vi "broadRvsTp.vi"(2 "# points":dbl=1023.0 format="%.2f", 3 "R_offset":dbl format="%.3f", 4 "Delta T":dbl=1.15 format="%.3f", 5 "T mean":dbl=2.35 format="%.3f", 6 "T max":dbl=12.0 format="%.2f", 7 "T min":dbl format="%.2f", 8 "n norm?":u8=7, 9 "?":dbl[][](array[numeric])=[[0.478, 1.52], [0.813, 3.56], [1.165, 8.95], [1.47, 17.94], [1.82, 37.19], [2.1, 58.77], [2.5, 82.04], [3.0, 101.16], [3.5, 98.64], [4.2, 100.83], [5.0, 101.87], [6.0, 94.77], [7.0, 85.01], [8.0, 75.33], [9.0, 67.49], [10.0, 60.86], [11.0, 56.85]] format="%.2f") -> (0 "sumsqu":dbl format="%.6f", 1 "r_0":dbl format="%.2f")   [LabVIEW 2018]
uses:
  <vilib>/Analysis/NI_AALPro.lvlib
  <vilib>/gmath/NI_Gmath.lvlib
  <vilib>/Analysis/NI_AALBase.lvlib
panel:
  in  "save fit?":bool
  in  "format":string="%.6e"
  out "?":dbl[](array[numeric]) format="%.2f"
  in  "R_offset copy":dbl format="%.3f"
  out "?":dbl=2045.0 format="%.2f"
  out "n":u32=17
  out "?":cluster{dbl[], dbl[]}[](graph)
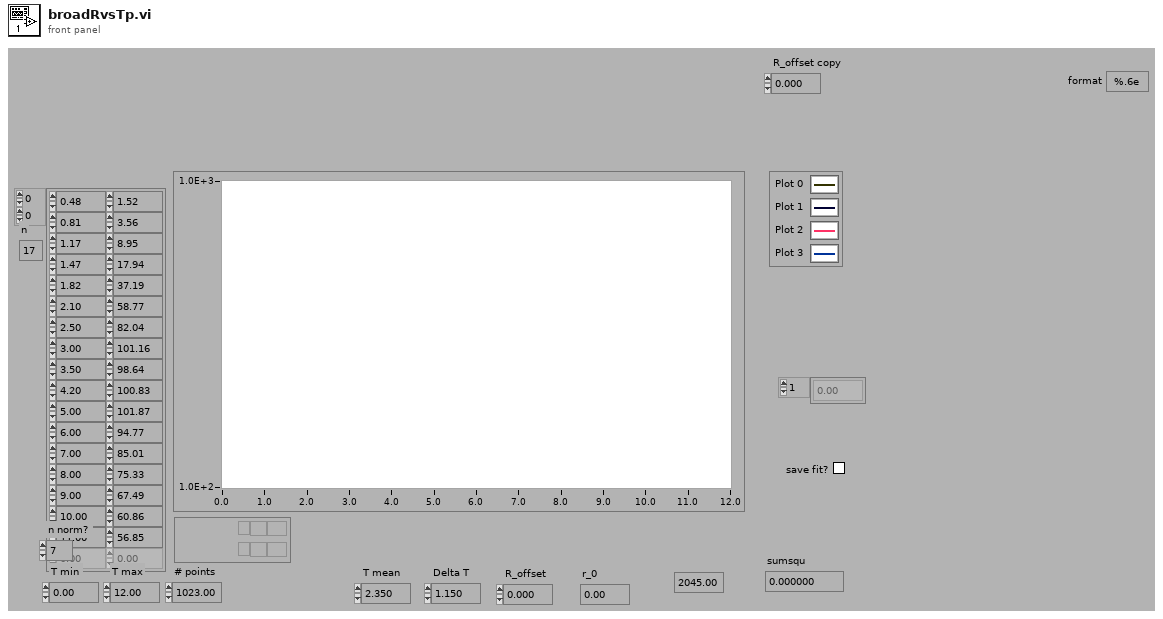
[diagram p1: front panel]
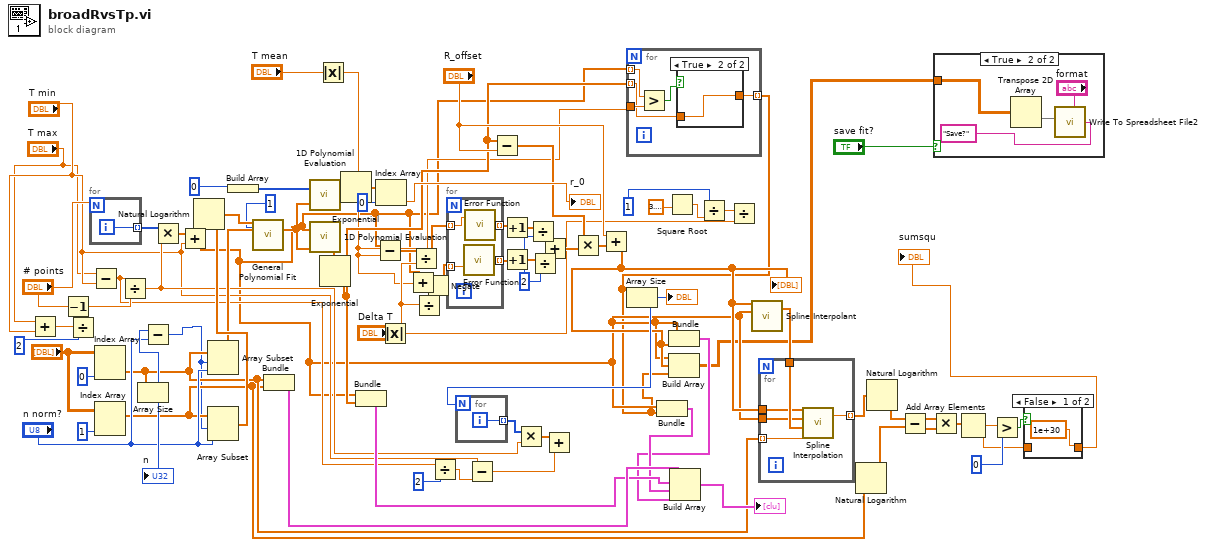
[diagram p0: block diagram]
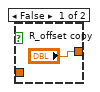
[diagram p3: hidden frame]
diagram:
  w24 = 2
  n1 = Add(x="T max", y="T min") -> (x+y=w53:dbl)
  n2 = Decrement(x="# points") -> (x-1=w76:dbl)
  n3 = Divide(x=w53, y=2) -> ()  [unwired: 1 out]
  n4 = for {
    N: "# points" -> [_]
    tunnel: [w82] -> w75 mode=indexing
    i -> [w82]
  }
  n5 = Subtract(x="T max", y="T min") -> (x-y=w65:dbl)
  n6 = Index Array(array="?", index (col)=0) -> (element=w51:dbl[])  [unwired: 1 in]
  n7 = Index Array(array="?", index (col)=1) -> (element=w49:dbl[])  [unwired: 1 in]
  n8 = Divide(x=w65, y=w76) -> (x/y=w56:dbl)
  n9 = Array Size(array=w51) -> (size(s)=w78:i32)
  "n" <- w78
  n10 = Subtract(x=w78, y="n norm?") -> (x-y=w1:i32)
  n11 = Multiply(x=w75, y=w56) -> (x*y=w74:dbl[])
  n12 = Add(x=w74, y="T min") -> (x+y=w4:dbl[])
  n13 = Array Subset(array=w51, index=w1, length="n norm?") -> (w69:dbl[])
  n14 = Array Subset(array=w49, index=w1, length="n norm?") -> (w70:dbl[])
  n15 = Natural Logarithm(1:w70) -> (0:w34:dbl[])
  n16 = Build Array(0) -> (w38:i32[])
  n17 = call <vilib>:"General Polynomial Fit.vi"("Y"=w34, "polynomial order"=1, "X"=w69) -> ("Polynomial Coefficients"=w40:dbl[])  [unwired: 9 in, 3 out]
  n18 = Bundle(w51, w49) -> (w73:cluster{dbl[], dbl[]})  [unwired: 1 in]
  n19 = call <vilib>:"1D Polynomial Evaluation.vi"("Coefficients: a"=w40, "X"=w38) -> ("Y"=w36:dbl[])  [unwired: 1 out]
  n20 = call <vilib>:"1D Polynomial Evaluation.vi"("Coefficients: a"=w40, "X"=w4) -> ("Y"=w17:dbl[])  [unwired: 1 out]
  n21 = Absolute Value(x="T mean") -> (abs(x)=w7:dbl)
  n22 = Exponential(1:w17) -> (0:w16:dbl[])
  n23 = Exponential(1:w36) -> (0:w33:dbl[])
  n24 = Bundle(w4, w16) -> (w72:cluster{dbl[], dbl[]})  [unwired: 1 in]
  n25 = Subtract(x=w4, y=w7) -> (x-y=w28:dbl[])
  n26 = Index Array(array=w33, index=0) -> (element=→"r_0":dbl)
  n27 = Absolute Value(x="Delta T") -> (abs(x)=w8:dbl)
  n28 = Add(x=w4, y=w7) -> (x+y=w14:dbl[])
  n29 = Divide(x=w28, y=w8) -> (x/y=w27:dbl[])
  n30 = Divide(x=w14, y=w8) -> (x/y=w12:dbl[])
  n31 = Negate(x=w12) -> (-x=w10:dbl[])
  n32 = Divide(x=w65, y=2) -> (x/y=w64:dbl)
  n33 = for {
    tunnel: w10 -> [w86] mode=indexing
    tunnel: w27 -> [w85] mode=indexing
    tunnel: [w84] -> w26 mode=indexing
    tunnel: [w83] -> w25 mode=indexing
    n34 = call <vilib>:"Error Function.vi"("x"=w86) -> ("erf(x)"=w83:dbl)  [unwired: 2 in]
    n35 = call <vilib>:"Error Function.vi"("x"=w85) -> ("erf(x)"=w84:dbl)  [unwired: 2 in]
  }
  n36 = Subtract(x="T min", y=w64) -> (x-y=w63:dbl)
  n37 = Subtract(x=w16, y="R_offset") -> (x-y=w20:dbl[])
  n38 = Increment(x=w26) -> (x+1=w22:dbl[])
  n39 = Increment(x=w25) -> (x+1=w23:dbl[])
  n40 = Divide(x=w22, y=w24) -> (x/y=w11:dbl[])
  n41 = Divide(x=w23, y=w24) -> (x/y=w21:dbl[])
  n42 = Add(x=w11, y=w21) -> (x+y=w9:dbl[])
  n43 = Multiply(x=w20, y=w9) -> (x*y=w19:dbl[])
  n44 = Add(x="R_offset", y=w19) -> (x+y=w5:dbl[])
  "?" <- w5
  n45 = for {
    tunnel: w16 -> [w88] mode=indexing
    tunnel: w4 -> [w90] mode=indexing
    tunnel: w7 -> [w91]
    tunnel: [w87] -> w2 mode=indexing
    n46 = Greater?(x=w90, y=w91) -> (0:w89:bool)
    n47 = case shown="True" w89 {
      tunnel: w88 -> [_ w93]
      tunnel: ["R_offset copy" w93] -> w87
      frame False {
      }
      frame True {
      }
    }
  }
  n48 = Array Size(array=w2) -> (size(s)=w68:i32)
  "?" <- w68
  n49 = for {
    N: w68 -> [_]
    tunnel: [w94] -> w67 mode=indexing
    i -> [w94]
  }
  n50 = Multiply(x=w67, y=w56) -> (x*y=w62:dbl[])
  n51 = Add(x=w62, y=w63) -> ()  [unwired: 1 out]
  n52 = Bundle(w4, w2) -> (w61:cluster{dbl[], dbl[]})  [unwired: 1 in]
  n53 = Square Root(x=3.141592653589793) -> (sqrt(x)=w59:dbl)
  n54 = Bundle(w4, w5) -> (w55:cluster{dbl[], dbl[]})  [unwired: 1 in]
  n55 = Build Array(w4, w5, w2) -> (w3:dbl[][])
  n56 = Build Array(w73, w72, w61, w55) -> (→"?":cluster{dbl[], dbl[]}[])
  n57 = Divide(x=1, y=w59) -> (x/y=w57:dbl)
  n58 = Divide(x=w57, y=w8) -> ()  [unwired: 1 out]
  n59 = call <vilib>:"Spline Interpolant.vi"("X"=w4, "Y"=w5) -> ("Interpolant"=w52:dbl[])  [unwired: 2 in, 1 out]
  n60 = for {
    tunnel: w52 -> [w99]
    tunnel: w51 -> [w98] mode=indexing
    tunnel: w4 -> [w97]
    tunnel: w5 -> [w96]
    tunnel: [w95] -> w50 mode=indexing
    n61 = call <vilib>:"Spline Interpolation.vi"("x value"=w98, "Interpolant"=w99, "X"=w97, "Y"=w96) -> ("interpolation value"=w95:dbl)  [unwired: 1 out]
  }
  n62 = Natural Logarithm(1:w49) -> (0:w45:dbl[])
  n63 = Natural Logarithm(1:w50) -> (0:w46:dbl[])
  n64 = Subtract(x=w46, y=w45) -> (x-y=w48:dbl[])
  n65 = Multiply(x=w48, y=w48) -> (x*y=w47:dbl[])
  n66 = case shown="True" "save fit?" {
    tunnel: w3 -> [_ w100]
    frame False {
    }
    frame True {
      n67 = Transpose 2D Array(2D array=w100) -> (transposed array=w102:dbl[][])
      n68 = call "Write To Spreadsheet File2.vi"("dialogue"="Save?", "format (%.3f)"="format", "2D data"=w102) -> ()  [unwired: 5 in, 1 out]
    }
  }
  n69 = Add Array Elements(numeric array=w47) -> (sum=w43:dbl)
  n70 = Greater?(x=w43, y=0) -> (0:w42:bool)
  n71 = case shown="False" w42 {
    tunnel: w43 -> [_ w105]
    tunnel: [1e+30 w105] -> w41
    frame False {
    }
    frame True {
    }
  }
  "sumsqu" <- w41
